vi "Set Pixel Data.vi"(8 "error in":errorcluster, 10 "Pixel Data":u8[](array[numeric]), 11 "Generic Image in":refnum<class "Generic Image.lvclass">) -> (0 "error out":errorcluster, 3 "Generic Image out":refnum<class "Generic Image.lvclass">)   [LabVIEW 2024, in "Generic Image.lvclass"]
uses:
  Generic Image.lvclass
  Generic Image.lvclass/Generic Image.ctl
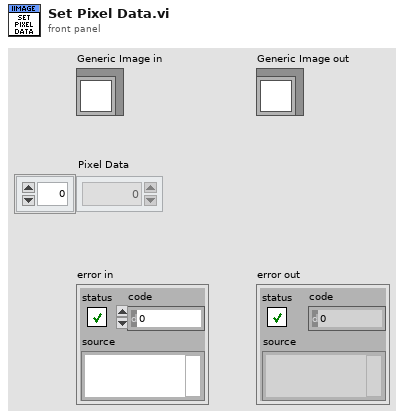
[diagram p1: front panel]
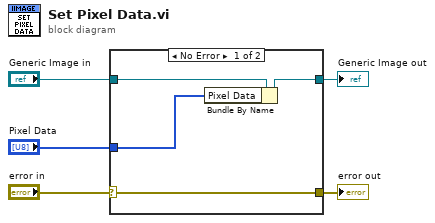
[diagram p0: block diagram]
diagram:
  n1 = case shown="No Error" "error in" {
    selector: "error in" -> [w6 w11]
    tunnel: "Generic Image in" -> [w9 w10]
    tunnel: [w8 w10] -> w4
    tunnel: "Pixel Data" -> [w7 _]
    tunnel: [w6 w11] -> w1
    frame No Error {
      n2 = Bundle By Name(cluster=w9, "Pixel Data"=w7) -> (w8:refnum<class "Generic Image.lvclass">)
    }
    frame Error {
    }
  }
  "error out" <- w1
  "Generic Image out" <- w4
